vi "LINC Convert Default Value.vi"(10 "default in":string) -> (2 "default out":string)   [LabVIEW 2018, in "STEPkgDriver_LINC.lvlib"]
uses:
  STEPkgDriver_LINC.lvlib
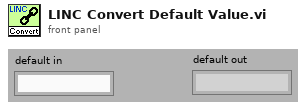
[diagram p1: front panel]
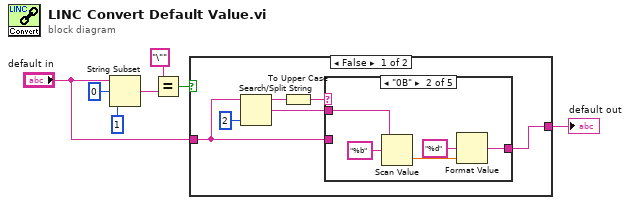
[diagram p0: block diagram]
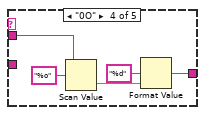
[diagram p4: hidden frame]
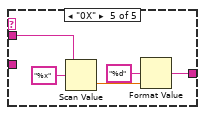
[diagram p5: hidden frame]
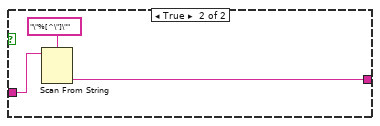
[diagram p6: hidden frame]
diagram:
  n1 = String Subset(string="default in", offset (0)=0, length (rest)=1 ("length (rest)")) -> (substring=w5:string)
  n2 = Equal?(x="\"", y=w5) -> (x = y?=w3:bool)
  n3 = case shown="False" w3 {
    tunnel: "default in" -> [w10 w32]
    tunnel: [w9 w31] -> w1
    frame False {
      n4 = Search/Split String(string=w10, offset (0)=2) -> (substring before match=w12:string, match + rest of string=w8:string)  [unwired: 1 in, 1 out]
      n5 = To Upper Case(1:w12) -> (0:w13:string)
      n6 = case shown="\"0B\"" w13 {
        tunnel: w10 -> [w14 _ _ _ _]
        tunnel: [w14 w16 w20 w22 w27] -> w9
        tunnel: w8 -> [_ w15 w20 w21 w26]
        frame Default {
        }
        frame "0B" {
          n7 = Scan Value(string=w15, format string="%b") -> (value=w18:dbl)  [unwired: 1 in, 1 out]
          n8 = Format Value(format string="%d", value (0)=w18) -> (output string=w16:string)  [unwired: 1 in]
        }
        frame "0D" {
        }
        frame "0O" {
          n9 = Scan Value(string=w21, format string="%o") -> (value=w24:dbl)  [unwired: 1 in, 1 out]
          n10 = Format Value(format string="%d", value (0)=w24) -> (output string=w22:string)  [unwired: 1 in]
        }
        frame "0X" {
          n11 = Scan Value(string=w26, format string="%x") -> (value=w29:dbl)  [unwired: 1 in, 1 out]
          n12 = Format Value(format string="%d", value (0)=w29) -> (output string=w27:string)  [unwired: 1 in]
        }
      }
    }
    frame True {
      n13 = Scan From String(format string="\"%[^\"]\"", input string=w32) -> (output 1=w31:string)  [unwired: 3 in, 3 out]
    }
  }
  "default out" <- w1
